vi "multiplier to color converter.vi"(2 "Multiplier select":T1) -> (6 "Multiplier color":u32(colorbox))   [LabVIEW 2018]
uses:
  multiplier--control.ctl
  Resistor Band Colors/Resistor Band Colors.lvlib
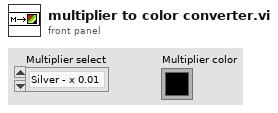
[diagram p1: front panel]
types:
  T1 = typedef "Multiplier--control.ctl" = enum16{"Silver - x 0.01", "Gold - x 0.1 ", "Black - x 1", "Brown - x 10", "Red - x 100", "Orange - x 1k", "Yellow - x 10k", "Green - 100k", "Blue - x 1M", "Violet - x10 M", "Grey - x 100M", "White - x 1G"}
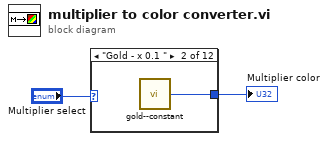
[diagram p0: block diagram]
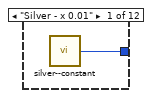
[diagram p2: hidden frame]
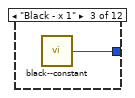
[diagram p3: hidden frame]
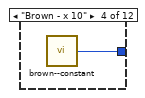
[diagram p4: hidden frame]
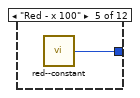
[diagram p5: hidden frame]
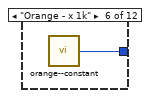
[diagram p6: hidden frame]
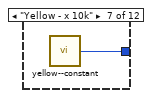
[diagram p7: hidden frame]
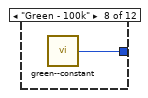
[diagram p8: hidden frame]
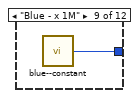
[diagram p9: hidden frame]
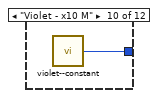
[diagram p10: hidden frame]
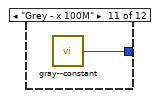
[diagram p11: hidden frame]
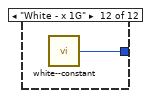
[diagram p12: hidden frame]
diagram:
  n1 = case shown="\"Gold - x 0.1 \"" "Multiplier select" {
    tunnel: [w3 w4 w5 w6 w7 w8 w9 w10 w11 w12 w13 w14] -> w1
    frame "Silver - x 0.01" {
      n2 = call "silver--constant.vi"() -> ("Silver"=w3:u32)  [unwired: 5 in]
    }
    frame "Gold - x 0.1 " {
      n3 = call "gold--constant.vi"() -> ("Gold"=w4:u32)  [unwired: 5 in]
    }
    frame "Black - x 1" {
      n4 = call "black--constant.vi"() -> ("Black"=w5:u32)  [unwired: 5 in]
    }
    frame "Brown - x 10" {
      n5 = call "brown--constant.vi"() -> ("Brown"=w6:u32)  [unwired: 5 in]
    }
    frame "Red - x 100" {
      n6 = call "red--constant.vi"() -> ("Red"=w7:u32)  [unwired: 5 in]
    }
    frame "Orange - x 1k" {
      n7 = call "orange--constant.vi"() -> ("Orange"=w8:u32)  [unwired: 5 in]
    }
    frame "Yellow - x 10k" {
      n8 = call "yellow--constant.vi"() -> ("Yellow"=w9:u32)  [unwired: 5 in]
    }
    frame "Green - 100k" {
      n9 = call "green--constant.vi"() -> ("Green"=w10:u32)  [unwired: 5 in]
    }
    frame "Blue - x 1M" {
      n10 = call "blue--constant.vi"() -> ("Blue"=w11:u32)  [unwired: 5 in]
    }
    frame "Violet - x10 M" {
      n11 = call "violet--constant.vi"() -> ("Violet"=w12:u32)  [unwired: 5 in]
    }
    frame "Grey - x 100M" {
      n12 = call "gray--constant.vi"() -> ("Gray"=w13:u32)  [unwired: 5 in]
    }
    frame "White - x 1G" {
      n13 = call "white--constant.vi"() -> ("White"=w14:u32)  [unwired: 5 in]
    }
  }
  "Multiplier color" <- w1
